vi "ClusterEscala.vi"() -> ()   [LabVIEW 2020]
panel:
  out "Cluster 2":T1 {"Gauge" scale=0.0..10000.0; "Tank" scale=0.0..10.0; "Thermometer" scale=0.0..100.0}
  out "x*y":cluster{dbl, dbl, dbl}
  in  "Cluster":T2
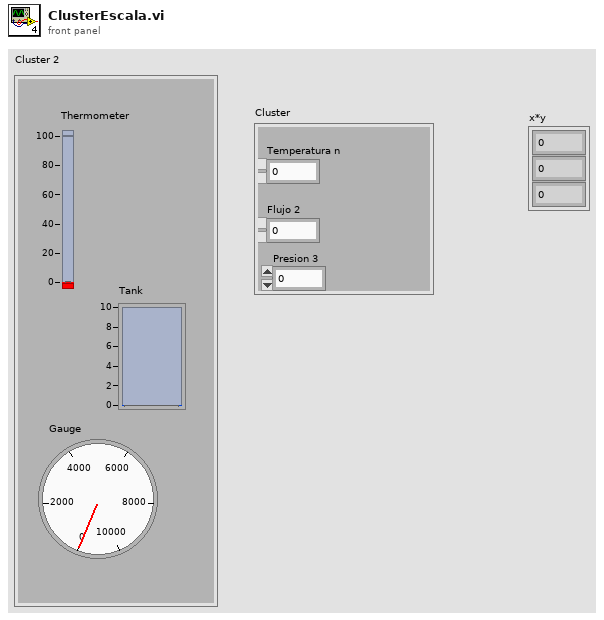
[diagram p1: front panel]
types:
  T1 = cluster{"Thermometer":dbl, "Tank":dbl, "Gauge":dbl}
  T2 = cluster{"Temperatura n":dbl, "Flujo 2":dbl, "Presion 3":dbl}
  T3 = cluster{"C/V°":dbl, "(I/s)/v Caudal":dbl, "(N/m^2)/V Presion":i32}
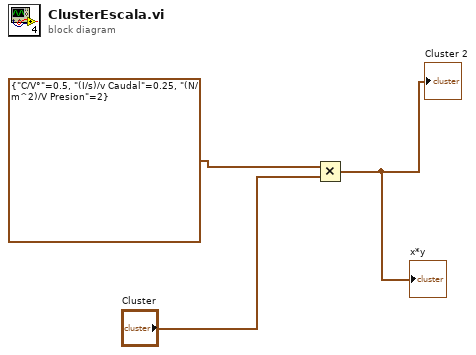
[diagram p0: block diagram]
diagram:
  n1 = Multiply(x=T3 {"C/V°"=0.5, "(I/s)/v Caudal"=0.25, "(N/m^2)/V Presion"=2}, y="Cluster") -> (x*y=→"x*y" →"Cluster 2":cluster{dbl, dbl, dbl})
